vi "FSM_Exec.vi"(8 "error in (no error)":errorcluster, 11 "FSM in":refnum<class "FSM.lvclass">) -> (0 "error out":errorcluster, 1 "current state":string, 3 "FSM out":refnum<class "FSM.lvclass">)   [LabVIEW 2021, in "FSM.lvclass"]
doc: "Run the Finite State Machine(FSM).\n\nAuthor: J. Camilo Gomez C."
uses:
  FSM.lvclass
  FSM.lvclass/FSM.ctl
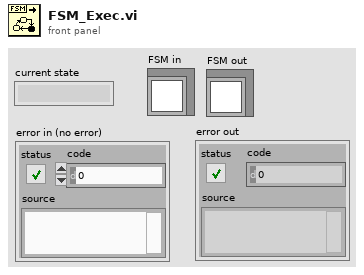
[diagram p1: front panel]
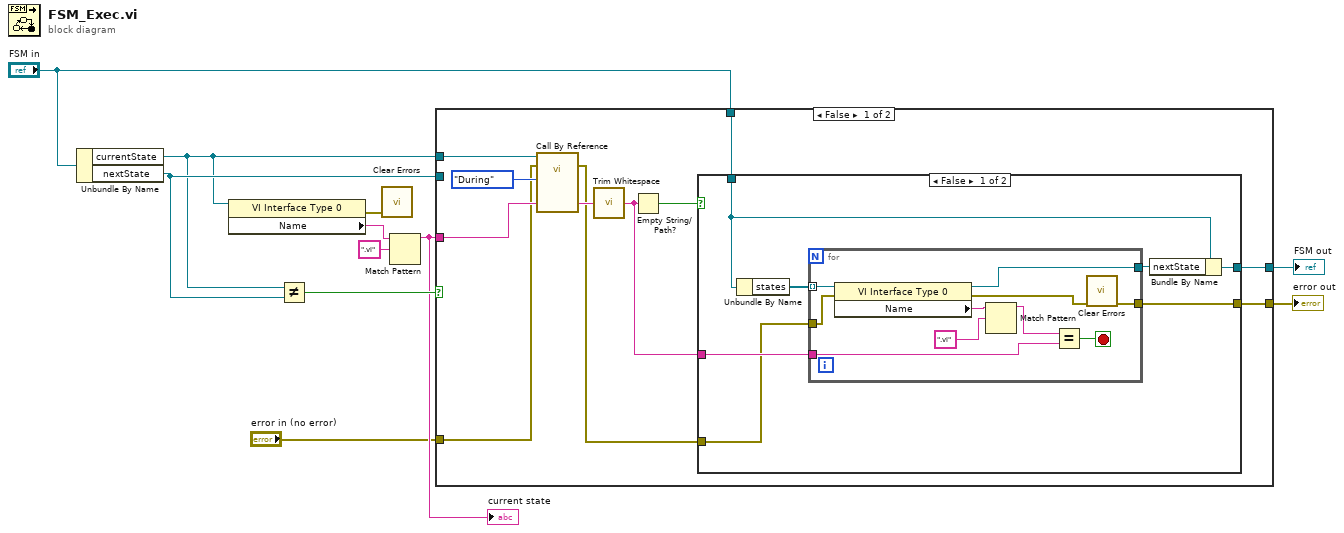
[diagram p0: block diagram]
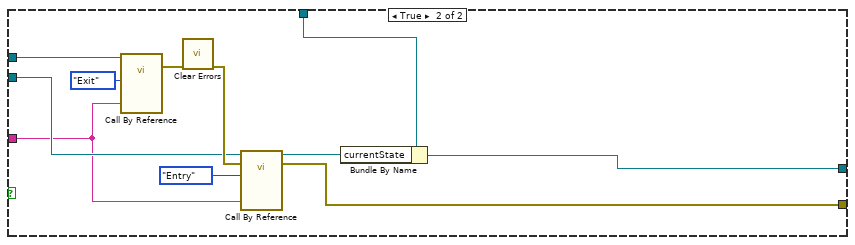
[diagram p3: hidden frame]
diagram:
  n1 = Unbundle By Name("FSM in") -> ("currentState"=w8:refnum<vi>, "nextState"=w10:refnum<vi>)
  n2 = property class="VI Interface Type 0"(reference=w8) -> (error out=w4:errorcluster, "Name"=w6:string)  [unwired: 1 in, 1 out]
  n3 = Not Equal?(x=w8, y=w10) -> (x != y?=w11:bool)
  n4 = call <vilib>:"Clear Errors.vi"("error in (no error)"=w4) -> ()  [unwired: 5 in, 2 out]
  n5 = Match Pattern(string=w6, regular expression=".vi") -> (before substring=w5:string)  [unwired: 1 in, 3 out]
  "current state" <- w5
  n6 = case shown="False" w11 {
    tunnel: w8 -> [w22 w51]
    tunnel: w10 -> [_ w47]
    tunnel: [w15 w46] -> w1
    tunnel: "FSM in" -> [w16 w45]
    tunnel: [w12 w43] -> w3
    tunnel: w5 -> [w20 w42]
    tunnel: "error in (no error)" -> [w14 _]
    frame False {
      n7 = call-by-ref "?"(reference=w22, error in=w14, "CurrentState"=w20, "Action"=enum16{"Entry", "During", "Exit"}."During") -> (error out=w13:errorcluster, "NextState"=w19:string)  [unwired: 9 in, 1 out]
      n8 = call <vilib>:"Trim Whitespace.vi"("string"=w19) -> ("trimmed string"=w17:string)  [unwired: 1 in]
      n9 = Empty String/Path?(string/path=w17) -> (empty?=w18:bool)
      n10 = case shown="False" w18 {
        tunnel: w17 -> [w29 _]
        tunnel: w16 -> [w26 w40]
        tunnel: [w25 w41] -> w15
        tunnel: w13 -> [w24 w41]
        tunnel: [w23 w40] -> w12
        frame False {
          n11 = Unbundle By Name(w26) -> ("states"=w28:refnum<vi>[])
          n12 = for {
            tunnel: w29 -> [w35]
            tunnel: w28 -> [w33] mode=indexing
            tunnel: [w32] -> w27
            tunnel: [w31] -> w25
            tunnel: w24 -> [w30]
            stop <- w34 stop-if-true
            n13 = property class="VI Interface Type 0"(reference=w33, error in=w30) -> (reference out=w32:refnum<vi>, error out=w39:errorcluster, "Name"=w38:string)
            n14 = Match Pattern(string=w38, regular expression=".vi") -> (before substring=w36:string)  [unwired: 1 in, 3 out]
            n15 = Equal?(x=w36, y=w35) -> (x = y?=w34:bool)
            n16 = call <vilib>:"Clear Errors.vi"("error in (no error)"=w39) -> ("error out"=w31:errorcluster)  [unwired: 5 in, 1 out]
          }
          n17 = Bundle By Name(cluster=w26, "nextState"=w27) -> (w23:refnum<class "FSM.lvclass">)
        }
        frame True {
        }
      }
    }
    frame True {
      n18 = call-by-ref "?"(reference=w51, "CurrentState"=w42, "Action"=enum16{"Entry", "During", "Exit"}."Exit") -> (error out=w50:errorcluster)  [unwired: 10 in, 2 out]
      n19 = call <vilib>:"Clear Errors.vi"("error in (no error)"=w50) -> ("error out"=w49:errorcluster)  [unwired: 5 in, 1 out]
      n20 = call-by-ref "?"(reference=w47, error in=w49, "CurrentState"=w42, "Action"=enum16{"Entry", "During", "Exit"}."Entry") -> (reference out=w44:refnum<vi>, error out=w46:errorcluster)  [unwired: 9 in, 1 out]
      n21 = Bundle By Name(cluster=w45, "currentState"=w44) -> (w43:refnum<class "FSM.lvclass">)
    }
  }
  "FSM out" <- w3
  "error out" <- w1
